vi "Initialize Thread UI.vi"(8 "error in (no error)":errorcluster, 10 "Thread Configuration":refnum<class "Configuration.lvclass">, 11 "Component UI in":refnum<class "Component UI.lvclass">) -> (0 "error out":errorcluster, 3 "Component UI out":refnum<class "Component UI.lvclass">)   [LabVIEW 2017, in "DSF Core.lvlib" / "Component UI.lvclass"]
uses:
  Component UI.lvclass
  Configuration/Configuration.lvclass
  Component UI.lvclass/Component UI.ctl
  User Interface/User Interface.lvclass
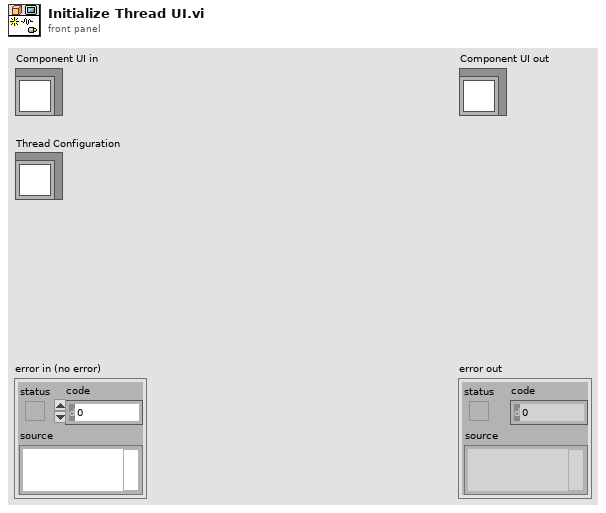
[diagram p1: front panel]
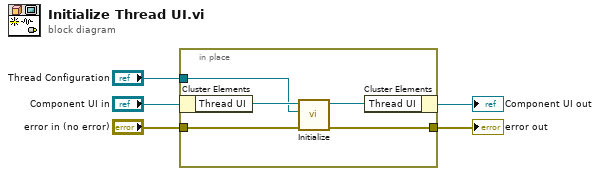
[diagram p0: block diagram]
diagram:
  n1 = in-place {
    in-place-border: "error in (no error)" -> [w8]
    in-place-border: [w7] -> w3
    in-place-border: "Thread Configuration" -> [w6]
    n2 = in-place-cluster #1("Component UI in") -> ("Thread UI"=w10:refnum<class "User Interface.lvclass">)
    n3 = call-dynamic "Initialize.vi"("error in (no error)"=w8, "Configuration"=w6, "User Interface in"=w10) -> ("error out"=w7:errorcluster, "User Interface out"=w9:refnum<class "User Interface.lvclass">)  [unwired: 7 in]
    n4 = in-place-cluster #1("Thread UI"=w9) -> (→"Component UI out":refnum<class "Component UI.lvclass">)
  }
  "error out" <- w3
